vi "Main.vi"() -> ()   [LabVIEW 2011]
uses:
  Controls/Signal Controls.ctl
  SlideEngine/SlideEngine.lvclass
  SlideEngine/SlideActions.ctl
panel:
  in  "2":enum32{"Page 1", "Page 2"}(tab)
  in  "Signal Controls 3":T1={"Frequency"=10.1, "Amplitude"=7.985611510791367, "Noise amplitude"=0.6, "Reset Button"=FALSE} {"Noise amplitude" scale=0.0..10.0; "Amplitude" scale=0.0..10.0; "Frequency" format="%#_g Hz"}
  in  "Tray 3 Lock":bool
  out "Locked? 3":bool
  in  "1":enum32{"Page 1", "Page 2"}(tab)
  in  "Signal Controls 2":T1={"Frequency"=10.1, "Amplitude"=7.985611510791367, "Noise amplitude"=0.6, "Reset Button"=FALSE} {"Noise amplitude" scale=0.0..10.0; "Amplitude" scale=0.0..10.0; "Frequency" format="%#_g Hz"}
  in  "Tray 2 Lock":bool
  out "Locked? 2":bool
  in  "0":enum32{"Page 1", "Page 2"}(tab)
  in  "Signal Controls":T1={"Frequency"=10.1, "Amplitude"=7.985611510791367, "Noise amplitude"=0.6, "Reset Button"=FALSE} {"Noise amplitude" scale=0.0..10.0; "Amplitude" scale=0.0..10.0; "Frequency" format="%#_g Hz"}
  in  "Tray 1 Lock":bool
  out "Locked? 1":bool
  out "Waveform Graph":dynamicdata(graph)
  in  "stop":bool
  # "Sliding Container Demo"
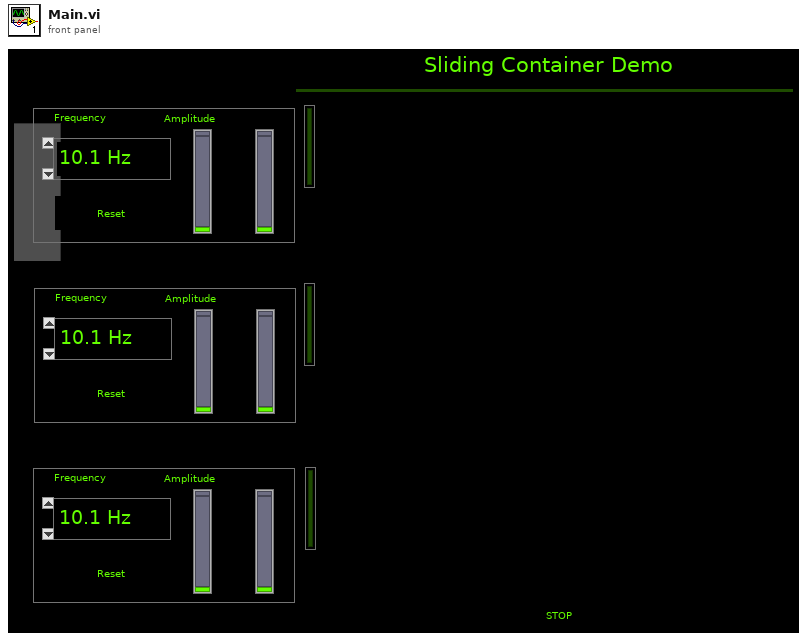
[diagram p1: front panel]
types:
  T1 = typedef "Signal Controls.ctl" = cluster{"Frequency":dbl, "Amplitude":dbl, "Noise amplitude":dbl, "Reset Button":bool}
  T2 = typedef "SlideActions.ctl" = enum16{"Left Open", "Left Close"}
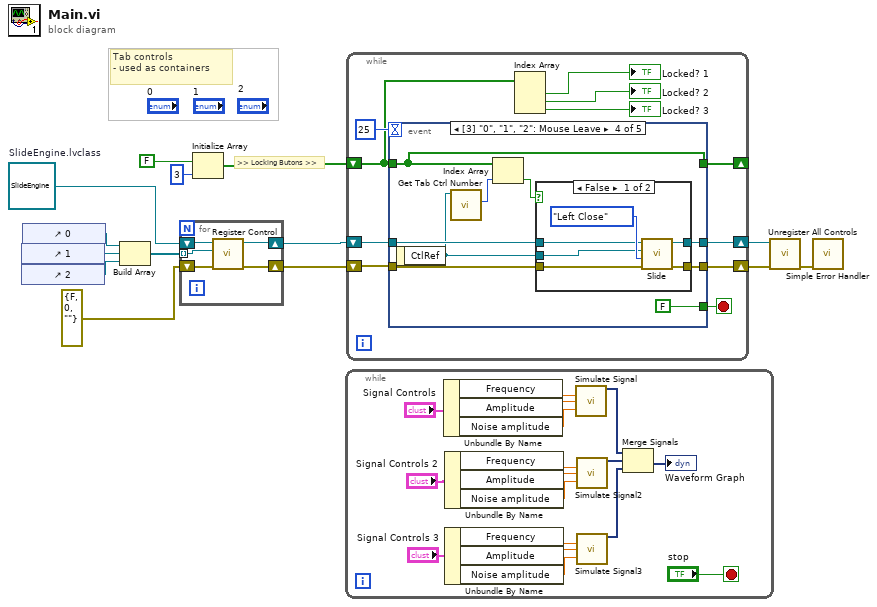
[diagram p0: block diagram]
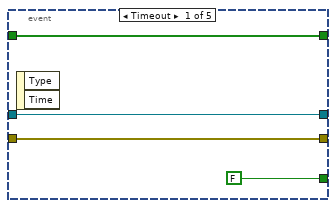
[diagram p2: hidden frame]
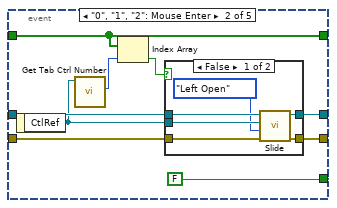
[diagram p3: hidden frame]
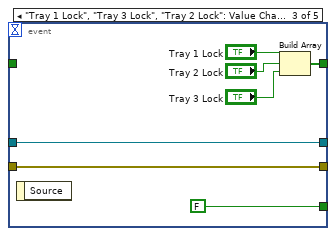
[diagram p5: hidden frame]
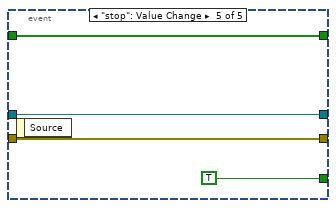
[diagram p7: hidden frame]
diagram:
  w2 = refnum<class "SlideEngine.lvclass"> refnum  # SlideEngine.lvclass
  # "Tab controls\n- used as containers"
  # ">> Locking Butons >>"
  n1 = control-ref of="1"() -> (w6:refnum<vi>)
  n2 = control-ref of="2"() -> (w5:refnum<vi>)
  n3 = control-ref of="0"() -> (w7:refnum<vi>)
  n4 = Build Array(w7, w6, w5) -> (w4:refnum<vi>[])
  n5 = for {
    shift-right: [w19] -> w3
    shift-left: w2 -> [w17]
    shift-right: [w18] -> w8
    shift-left: errorcluster {"status"=FALSE, "code"=0, "source"=""} ("error out") -> [w16]
    tunnel: w4 -> [w15] mode=indexing
    n6 = call "Register Control.vi"("error in (no error)"=w16, "Control to Register"=w15, "SlideEngine.lvclass In"=w17) -> ("error out"=w18:errorcluster, "SlideEngine.lvclass Out"=w19:refnum<class "SlideEngine.lvclass">)  [unwired: 7 out]
  }
  n7 = Initialize Array(FALSE, 3 ("dimension size")) -> (w12:bool[])
  n8 = while {
    stop <- "stop" stop-if-true
    n9 = Unbundle By Name("Signal Controls") -> ("Frequency"=w34:dbl, "Amplitude"=w35:dbl, "Noise amplitude"=w36:dbl)
    n10 = Unbundle By Name("Signal Controls 2") -> ("Frequency"=w32:dbl, "Amplitude"=w31:dbl, "Noise amplitude"=w30:dbl)
    n11 = Unbundle By Name("Signal Controls 3") -> ("Frequency"=w27:dbl, "Amplitude"=w28:dbl, "Noise amplitude"=w29:dbl)
    n12 = call "Simulate Signal"("Frequency"=w34, "Amplitude"=w35, "Noise amplitude"=w36) -> ("Sine with Uniform Noise"=w24:dynamicdata)  [unwired: 5 in, 7 out]
    n13 = call "Simulate Signal2"("Frequency"=w32, "Amplitude"=w31, "Noise amplitude"=w30) -> ("Sine with Uniform Noise"=w23:dynamicdata)  [unwired: 5 in, 7 out]
    n14 = call "Simulate Signal3"("Frequency"=w27, "Amplitude"=w28, "Noise amplitude"=w29) -> ("Sine with Uniform Noise"=w22:dynamicdata)  [unwired: 5 in, 7 out]
    n15 = Merge Signals(w24, w23, w22) -> (→"Waveform Graph":dynamicdata)
  }
  n16 = while {
    shift-right: [w43] -> _
    shift-left: w12 -> [w45]
    shift-right: [w39] -> w11
    shift-left: w8 -> [w40]
    shift-right: [w38] -> w10
    shift-left: w3 -> [w37]
    stop <- w47 stop-if-true
    n17 = event shown="[3] \"0\", \"1\", \"2\": Mouse Leave" {
      selector: _ -> [_ _ _ _ _]
      dyn-events: _ -> [_ _ _ _ _]
      timeout: 25 -> [_ _ _ _ _]
      tunnel: [FALSE FALSE FALSE FALSE TRUE] -> w47
      tunnel: w45 -> [w50 w60 _ w83 w96]
      tunnel: [w50 w60 w72 w83 w96] -> w43
      tunnel: w40 -> [w49 w54 w71 w78 w95]
      tunnel: [w49 w55 w71 w80 w95] -> w39
      tunnel: w37 -> [w48 w57 w69 w79 w93]
      tunnel: [w48 w56 w69 w81 w93] -> w38
      event Timeout {
        n18 = event-data() -> ()  [unwired: 3 out]
      }
      event "0", "1", "2": Mouse Enter {
        n19 = event-data() -> ("CtlRef"=w53:refnum<vi>)  [unwired: 1 out]
        n20 = call "Get Tab Ctrl Number.vi"("CtlRef"=w53) -> ("number"=w52:u32)  [unwired: 10 out]
        n21 = Index Array(array=w60, index=w52) -> (element=w59:bool)
        n22 = case shown="False" w59 {
          tunnel: w53 -> [w66 _]
          tunnel: w57 -> [w65 w68]
          tunnel: [w63 w68] -> w56
          tunnel: [w62 w67] -> w55
          tunnel: w54 -> [w61 w67]
          frame False {
            n23 = call "Slide.vi"("error in (no error)"=w61, "Action"=SlideActions."Left Open", "CtlRef"=w66, "SlideEngine.lvclass"=w65) -> ("error out"=w62:errorcluster, "SlideEngine.lvclass Out"=w63:refnum<class "SlideEngine.lvclass">)  [unwired: 6 out]
          }
          frame True {
          }
        }
      }
      event "Tray 1 Lock", "Tray 3 Lock", "Tray 2 Lock": Value Change {
        n24 = event-data() -> ()  [unwired: 2 out]
        n25 = Build Array("Tray 1 Lock", "Tray 2 Lock", "Tray 3 Lock") -> (w72:bool[])
      }
      event "0", "1", "2": Mouse Leave {
        n26 = event-data() -> ("CtlRef"=w77:refnum<vi>)  [unwired: 1 out]
        n27 = call "Get Tab Ctrl Number.vi"("CtlRef"=w77) -> ("number"=w76:u32)  [unwired: 10 out]
        n28 = Index Array(array=w83, index=w76) -> (element=w84:bool)
        n29 = case shown="False" w84 {
          tunnel: [w90 w92] -> w81
          tunnel: [w89 w91] -> w80
          tunnel: w79 -> [w87 w92]
          tunnel: w77 -> [w86 _]
          tunnel: w78 -> [w85 w91]
          frame False {
            n30 = call "Slide.vi"("error in (no error)"=w85, "Action"=enum16{"Left Open", "Left Close"}."Left Close", "CtlRef"=w86, "SlideEngine.lvclass"=w87) -> ("error out"=w89:errorcluster, "SlideEngine.lvclass Out"=w90:refnum<class "SlideEngine.lvclass">)  [unwired: 6 out]
          }
          frame True {
          }
        }
      }
      event "stop": Value Change {
        n31 = event-data() -> ()  [unwired: 2 out]
      }
    }
    n32 = Index Array(array=w45) -> (element #1=→"Locked? 1":bool, element #2=→"Locked? 2":bool, element #3=→"Locked? 3":bool)  [unwired: 3 in]
  }
  n33 = call "Unregister All Controls.vi"("error in (no error)"=w11, "SlideEngine.lvclass In"=w10) -> ("error out"=w9:errorcluster)  [unwired: 9 out]
  n34 = call <vilib>:"Simple Error Handler.vi"("error in (no error)"=w9) -> ()  [unwired: 1 in, 8 out]
